vi "Pay.vi"(8 "error in (no error)":errorcluster, 10 "Accoounts":T1(c390), 11 "ATransfer in":refnum<class "ATransfer.lvclass">) -> (0 "error out":errorcluster, 2 "Accoounts out":T1(c390), 3 "ATransfer out":refnum<class "ATransfer.lvclass">)   [LabVIEW 2020, in "ATransfer.lvclass"]
uses:
  ATransfer.lvclass
  ATransfer.lvclass/ATransfer.ctl
  IBasicAccount/IBasicAccount.lvclass
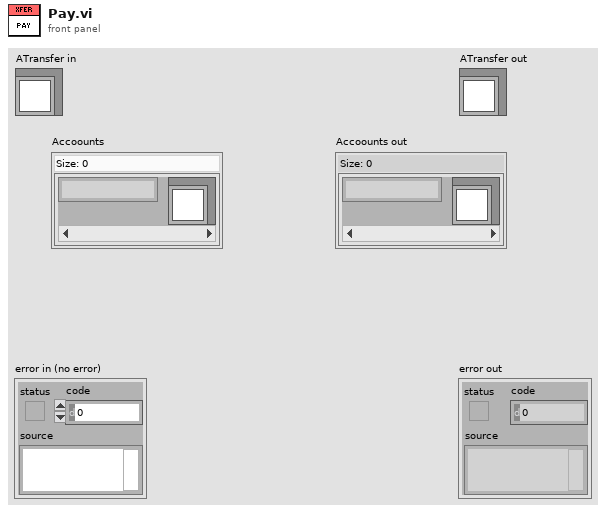
[diagram p1: front panel]
types:
  T1 = map{string, refnum<class "IBasicAccount.lvclass">}
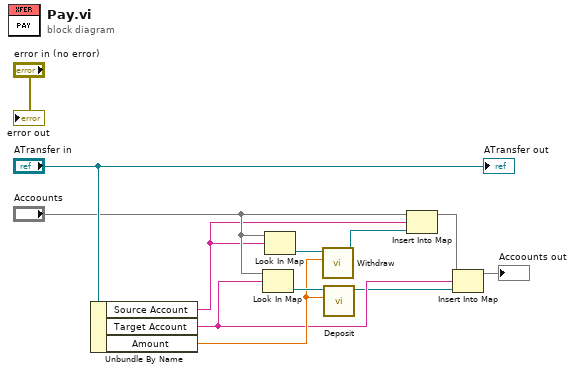
[diagram p0: block diagram]
diagram:
  n1 = Unbundle By Name("ATransfer in") -> ("Source Account"=w7:string, "Target Account"=w4:string, "Amount"=w9:dbl)
  n2 = Look In Map(map="Accoounts", key=w4) -> (value=w11:refnum<class "IBasicAccount.lvclass">)  [unwired: 1 in, 1 out]
  n3 = Look In Map(map="Accoounts", key=w7) -> (value=w10:refnum<class "IBasicAccount.lvclass">)  [unwired: 1 in, 1 out]
  n4 = call-dynamic "Withdraw.vi"("Amount"=w9, "IWithdrawable in"=w10) -> ("IWithdrawable out"=w6:refnum<class "IBasicAccount.lvclass">)  [unwired: 6 in, 3 out]
  n5 = call-dynamic "Deposit.vi"("Amount"=w9, "IDepositable in"=w11) -> ("IDepositable out"=w3:refnum<class "IBasicAccount.lvclass">)  [unwired: 7 in, 2 out]
  n6 = Insert Into Map(map in="Accoounts", key=w7, value=w6) -> (map out=w5:T1)  [unwired: 2 out]
  n7 = Insert Into Map(map in=w5, key=w4, value=w3) -> (map out=→"Accoounts out":T1)  [unwired: 2 out]
  "error out" <- "error in (no error)"
  "ATransfer out" <- "ATransfer in"
